vi "HornScan_Recipe_Sub_Vi.vi"(0 "connection ID":refnum<k5>, 4 "error in (no error)":errorcluster, 6 "SetDigitalTuneWithHornScan":u16, 7 "Receipe Msg ID":u32, 8 "Start Frequency":u32, 11 "Receipe Message length":u32, 12 "Max Current":u16, 13 "Max Amplitude":u16, 14 "Frequency Step":u16, 15 "Time Delay":u16, 16 "Stop Frequency":u32, 17 "Response ID":i32) -> (20 "String":string=" Success", 21 "connection ID":refnum<k5>, 27 "error out":errorcluster)   [LabVIEW 2017]
panel:
  out "bytes written":i32
  # "OUTPUT"
  # "/* Limits for 20 khz horn */\n#define HORN_START_FREQ_MIN_20KHZ 19450\n#define HORN_STOP_FREQ_MAX_20KHZ 20449\n#define HORN_FREQ_STEP_MAX_20KHZ 1000\n \n/* Limits for 30khz horn */\n#define HORN_START_FREQ_MIN_30KHZ 29250\n#define HORN_STOP_FREQ_MAX_30KHZ 30749\n#define HORN_FREQ_STEP_MAX_30KHZ 1500\n \n/* Limits for 40 khz horn */\n#define HORN_START_FREQ_MIN_40KHZ 39000\n#define HORN_STOP_FREQ_MAX_40KHZ 40999\n#define HORN_FREQ_STEP_MAX_40KHZ 2000"
  # "INPUT"
  # "Info:"
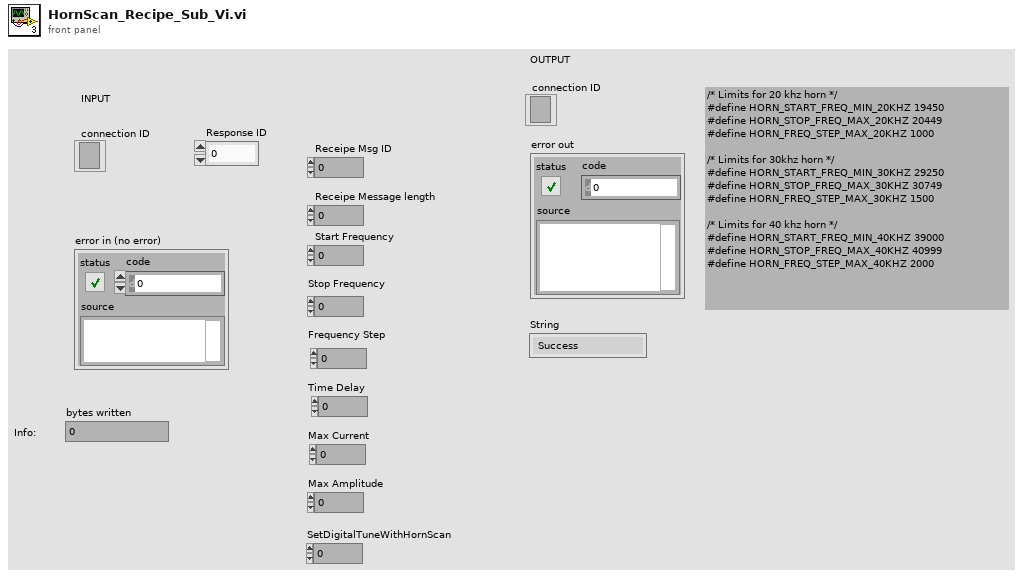
[diagram p1: front panel]
types:
  T1 = enum16{"big-endian, network order", "native, host order", "little-endian"}
  T2 = cluster{"SetDigitalTuneWithHornScan":u16, "Max Amplitude":u16, "Max Current":u16, "Time Delay":u16, "Frequency Step":u16, "Stop Frequency":u32, "Start Frequency":u32, "Receipe Message length":u32, "Receipe Msg ID":u32}
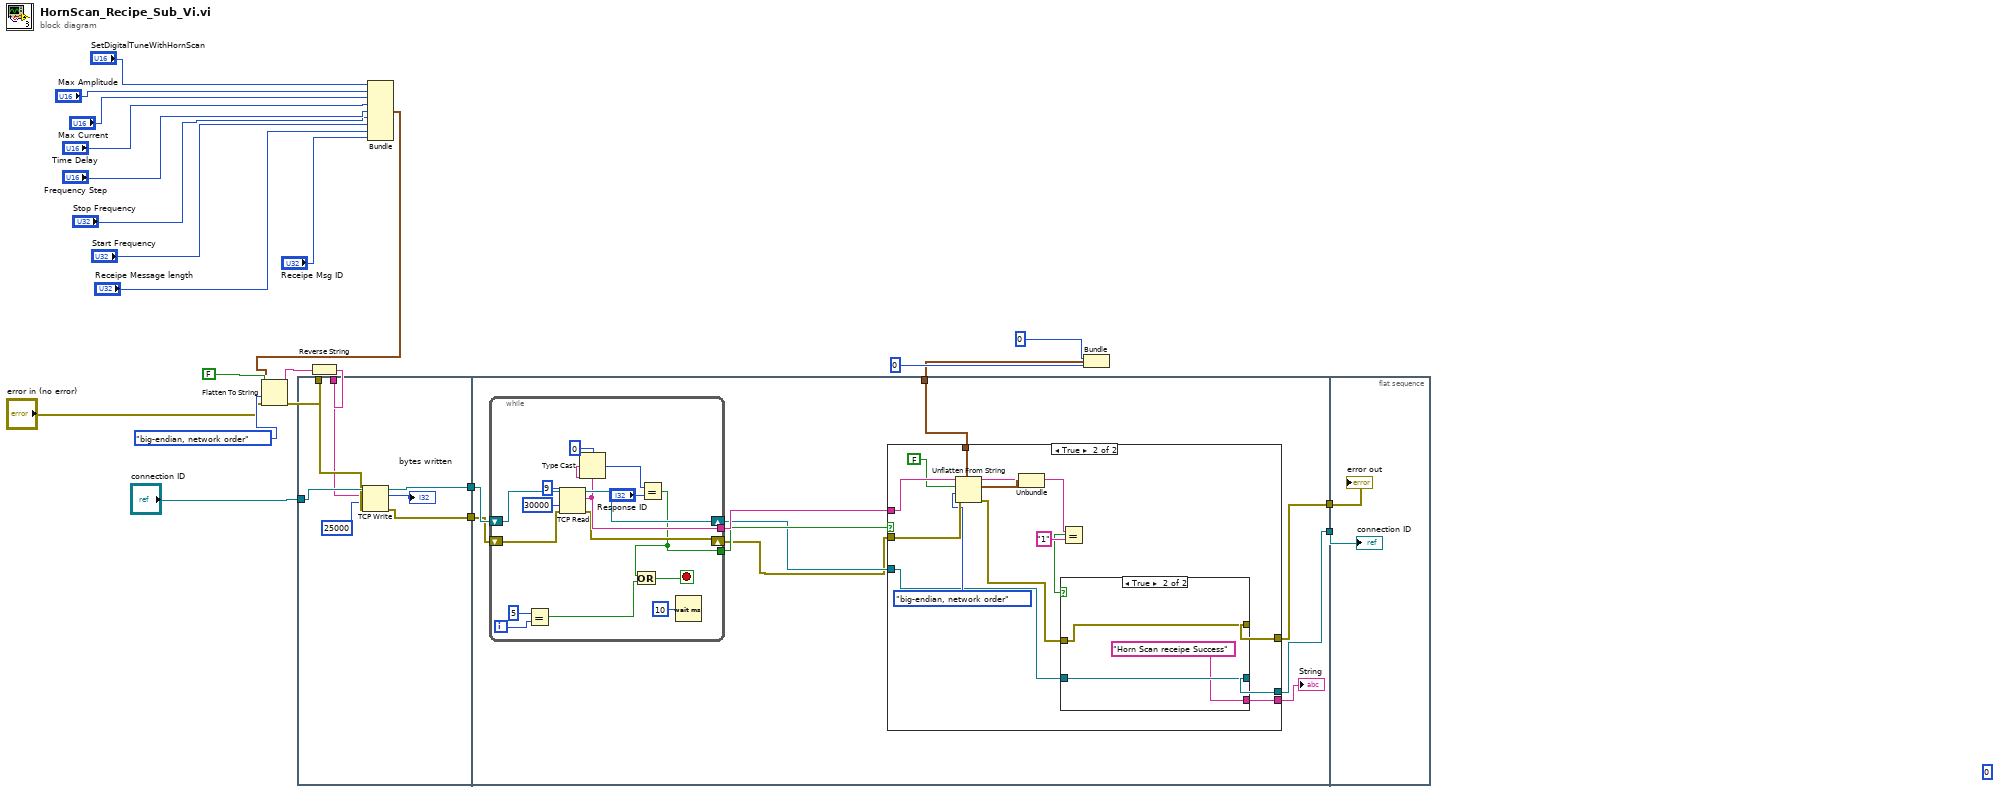
[diagram p0: block diagram]
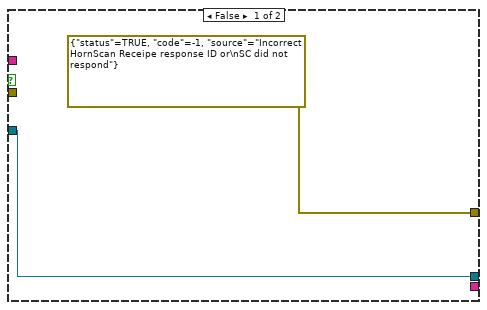
[diagram p2: hidden frame]
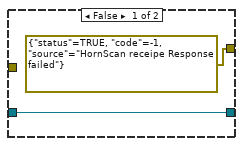
[diagram p3: hidden frame]
diagram:
  (unwired) u8 0
  n1 = flat-sequence {
    tunnel: "connection ID" -> [w31]
    tunnel: w20 -> [w30]
    tunnel: w18 -> [w29]
    tunnel: [w26] -> w2
    tunnel: [w25] -> w1
    tunnel: [w37] -> w24
    tunnel: [w38] -> w23
    tunnel: w11 -> [w39]
    tunnel: w2 -> [w35]
    tunnel: w1 -> [w34]
    tunnel: w24 -> [w79]
    tunnel: w23 -> [w80]
    frame #0 {
      n2 = TCP Write(connection ID=w31, data in=w29, error in (no error)=w30, 9:25000 ("timeout ms (25000)")) -> (connection ID out=w26:refnum<k5>, bytes written=→"bytes written":i32, error out=w25:errorcluster)
    }
    frame #1 {
      n3 = while {
        tunnel: [w77] -> w41
        shift-right: [w78] -> w33
        shift-left: w35 -> [w66]
        shift-right: [w74] -> w32
        shift-left: w34 -> [w65]
        tunnel: [w73] -> w40
        i -> [w72]
        stop <- w69 stop-if-true
        n4 = Equal?(x=5, y=w72) -> (x = y?=w70:bool)
        n5 = TCP Read(connection ID=w66, bytes to read=9, error in (no error)=w65, 9:30000 ("timeout ms (25000)")) -> (connection ID out=w78:refnum<k5>, data out=w77:string, error out=w74:errorcluster)  [unwired: 1 in]
        n6 = Type Cast(type=u8 0, x=w77) -> (*(type *) &x=w75:u8)
        n7 = Equal?(x=w75, y="Response ID") -> (x = y?=w73:bool)
        n8 = Or(x=w73, y=w70) -> (x .or. y?=w69:bool)
        n9 = Wait (ms)(milliseconds to wait=u32 10) -> ()  [unwired: 1 out]
      }
      n10 = case shown="True" w40 {
        tunnel: w32 -> [_ w57]
        tunnel: w41 -> [_ w56]
        tunnel: w33 -> [w42 w45]
        tunnel: w39 -> [_ w52]
        tunnel: [errorcluster {"status"=TRUE, "code"=-1, "source"="Incorrect HornScan Receipe response ID or\nSC did not respond"} ("error constant") w48] -> w38
        tunnel: [w42 w46] -> w37
        tunnel: [_ w44] -> w36
        frame False {
        }
        frame True {
          n11 = Unflatten From String(type=w52, binary string=w56, data includes array or string size? (T)=FALSE, byte order (0:big-endian, network order)=T1."big-endian, network order", error in (no error)=w57) -> (rest of the binary string=w51:string, value=w53:cluster{i32, i32}, error out=w49:errorcluster)
          n12 = Unbundle(w53) -> ()  [unwired: 2 out]
          n13 = Equal?(x=w51, y="1") -> (x = y?=w47:bool)
          n14 = case shown="True" w47 {
            tunnel: w49 -> [_ w62]
            tunnel: [errorcluster {"status"=TRUE, "code"=-1, "source"="HornScan receipe Response failed"} ("error constant") w62] -> w48
            tunnel: w45 -> [w58 w61]
            tunnel: [w58 w61] -> w46
            tunnel: [_ "Horn Scan receipe Success"] -> w44
            frame False {
            }
            frame True {
            }
          }
        }
      }
      "String" <- w36
    }
    frame #2 {
      "connection ID" <- w79
      "error out" <- w80
    }
  }
  n15 = Bundle("SetDigitalTuneWithHornScan"="SetDigitalTuneWithHornScan", "Max Amplitude"="Max Amplitude", "Max Current"="Max Current", "Time Delay"="Time Delay", "Frequency Step"="Frequency Step", "Stop Frequency"="Stop Frequency", "Start Frequency"="Start Frequency", "Receipe Message length"="Receipe Message length", "Receipe Msg ID"="Receipe Msg ID") -> (w14:T2)  [unwired: 1 in]
  n16 = Flatten To String(anything=w14, prepend array or string size? (T)=FALSE, byte order (0:big-endian, network order)=T1."big-endian, network order", error in (no error)="error in (no error)") -> (data string=w19:string, error out=w20:errorcluster)  [unwired: 1 out]
  n17 = Reverse String(1:w19) -> (0:w18:string)
  n18 = Bundle(0, 0) -> (w11:cluster{i32, i32})  [unwired: 1 in]
